vi "NoITsn.vi"(7 "S/N":string, 8 "localDataBase?":bool, 10 "P/N":string, 11 "DBSet":T1) -> (0 "shi jin zhi Sn":string, 1 "Customer data":string, 2 "未经进制转换的sn(客户 jin zhi sn)":string, 3 "show_date":timestamp, 4 "strFSN 原始SN(Include #)":string, 5 "输出的label内容":string="CN0T11GF7720661R7005A00#20160127#7005", 6 "result?":bool, 9 "status":bool)   [LabVIEW 2011]
panel:
  out "result":string[](array[string])
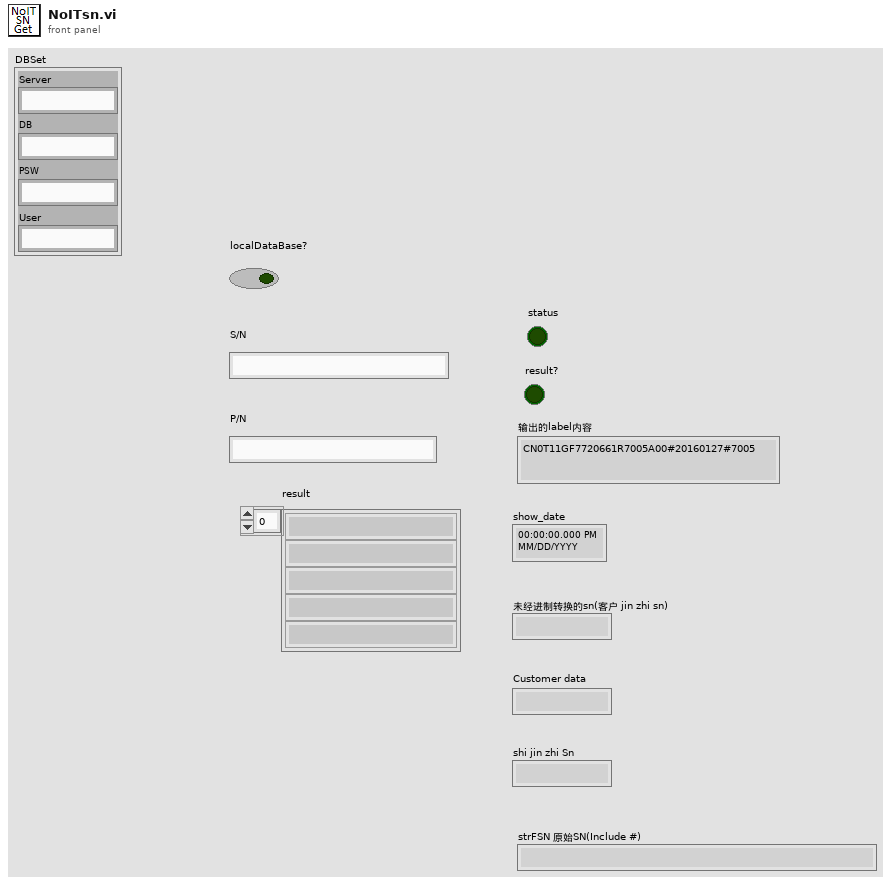
[diagram p1: front panel]
types:
  T1 = cluster{"Server":string, "DB":string, "PSW":string, "User":string}
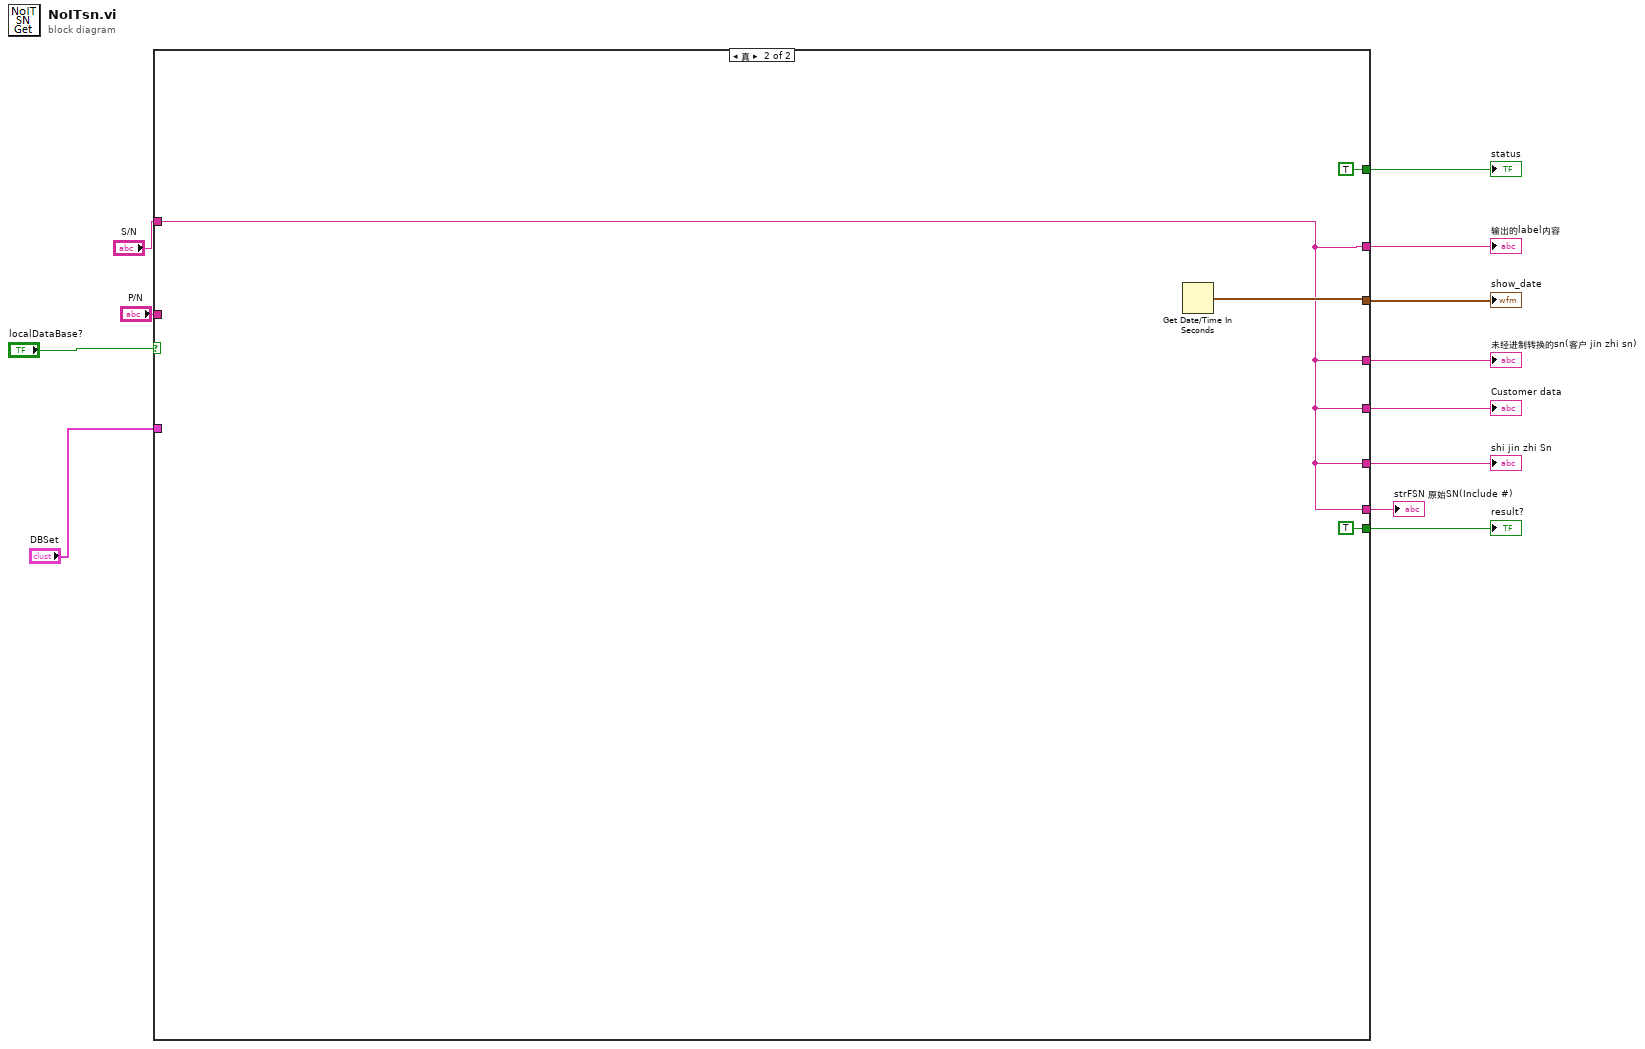
[diagram p0: block diagram]
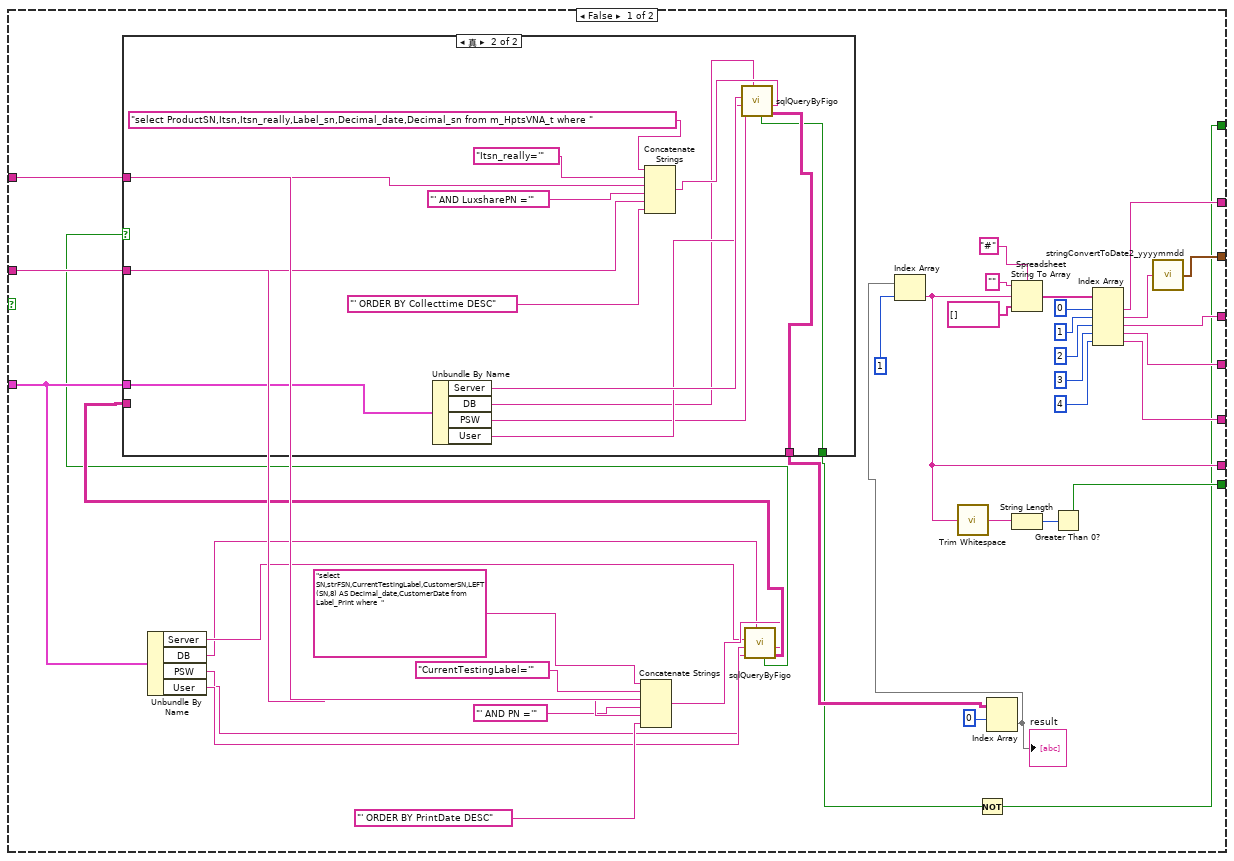
[diagram p2: hidden frame]
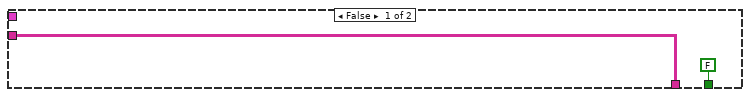
[diagram p3: hidden frame]
diagram:
  n1 = case shown="真" "localDataBase?" {
    tunnel: "S/N" -> [w28 w68]
    tunnel: "P/N" -> [w27 _]
    tunnel: [w29 TRUE] -> w10
    tunnel: [w42 w68] -> w9
    tunnel: [w40 w69] -> w8
    tunnel: [w39 w68] -> w7
    tunnel: [w35 w68] -> w6
    tunnel: [w34 w68] -> w5
    tunnel: [w31 TRUE] -> w4
    tunnel: [w30 w68] -> w2
    tunnel: "DBSet" -> [w19 _]
    frame False {
      n2 = Unbundle By Name(w19) -> ("Server"=w18:string, "DB"=w15:string, "PSW"=w16:string, "User"=w17:string)
      n3 = Concatenate Strings("select SN,strFSN,CurrentTestingLabel,CustomerSN,LEFT(SN,8) AS Decimal_date,CustomerDate from Label_Print where  " ("columns"), "CurrentTestingLabel='" ("字符串"), w28, "' AND PN ='" ("字符串"), w27, "' ORDER BY PrintDate DESC" ("字符串")) -> (w20:string)
      n4 = call "sqlQueryByFigo.vi"("SQL"=w20, "DATABASE"=w15, "password"=w16, "user id"=w17, "Server"=w18) -> ("查询数据"=w21:string[][], "query status"=w14:bool)  [unwired: 5 in]
      n5 = case shown="真" w14 {
        tunnel: w28 -> [_ w65]
        tunnel: w27 -> [_ w64]
        tunnel: [w53 w60] -> w24
        tunnel: w19 -> [_ w61]
        tunnel: w21 -> [w53 _]
        tunnel: [FALSE ("query status") w58] -> w13
        frame False {
        }
        frame True {
          n6 = Unbundle By Name(w61) -> ("Server"=w57:string, "DB"=w54:string, "PSW"=w55:string, "User"=w56:string)
          n7 = Concatenate Strings("select ProductSN,Itsn,Itsn_really,Label_sn,Decimal_date,Decimal_sn from m_HptsVNA_t where " ("columns"), "Itsn_really='" ("字符串"), w65, "' AND LuxsharePN ='" ("字符串"), w64, "' ORDER BY Collecttime DESC" ("字符串")) -> (w59:string)
          n8 = call "sqlQueryByFigo.vi"("SQL"=w59, "DATABASE"=w54, "password"=w55, "user id"=w56, "Server"=w57) -> ("查询数据"=w60:string[][], "query status"=w58:bool)  [unwired: 5 in]
        }
      }
      n9 = Not(x=w13) -> (.not. x?=w29:bool)
      n10 = Index Array(array=w24, index (row)=0 ("索引 (行)")) -> (element=w50:string[])  [unwired: 1 in]
      "result" <- w50
      n11 = Index Array(array=w50, index=1 ("索引")) -> (element=w30:string)
      n12 = call <vilib>:"Trim Whitespace.vi"("string"=w30) -> ("trimmed string"=w33:string)  [unwired: 1 in]
      n13 = Spreadsheet String To Array(delimiter (Tab)="#" ("分隔符(Tab)"), format string="" ("格式字符串"), spreadsheet string=w30, array type (2D Dbl)=string[] []) -> (array=w46:string[])
      n14 = String Length(string=w33) -> (length=w32:i32)
      n15 = Greater Than 0?(x=w32) -> (x > 0?=w31:bool)
      n16 = Index Array(array=w46, index #1=0 ("索引"), index #2=1 ("索引"), index #3=2 ("索引"), index #4=3 ("索引"), index #5=4 ("索引")) -> (element #1=w42:string, element #2=w41:string, element #3=w39:string, element #4=w35:string, element #5=w34:string)
      n17 = call "stringConvertToDate2_yyyymmdd.vi"("input_str_yyyymmdd"=w41) -> ("show_date"=w40:timestamp)
    }
    frame True {
      n18 = Get Date/Time In Seconds() -> (seconds since 1Jan1904=w69:timestamp)
    }
  }
  "status" <- w10
  "输出的label内容" <- w9
  "show_date" <- w8
  "未经进制转换的sn(客户 jin zhi sn)" <- w7
  "Customer data" <- w6
  "shi jin zhi Sn" <- w5
  "result?" <- w4
  "strFSN 原始SN(Include #)" <- w2
